vi "Load.vi"(6 "replace if found? (F)":bool, 8 "error in (no error)":errorcluster, 9 "create file if necessary? (T)":bool=TRUE, 10 "configuration file path":path, 11 "DSF Configuration Reference in":T1) -> (0 "error out":errorcluster, 1 "file replaced?":bool, 2 "file created?":bool, 3 "DSF Configuration Reference out":T1)   [LabVIEW 2017, in "Data Sharing Framework Core.lvlib" / "Data Sharing Framework Configuration.lvlib"]
uses:
  Data Sharing Framework Configuration.lvlib
  Controls/Session/DSF Configuration Reference.ctl
  Controls/DSF File Format/Internal.DSF Configuration.ctl
  Public/Controls/DSF Version Info.ctl
  Controls/DSF File Format/Internal.DSF Plugin with ID.ctl
  Controls/DSF File Format/Internal.DSF Plugin Info.ctl
  Public/Controls/DSF Timing Info.ctl
  Controls/DSF File Format/Internal.DSF Group with ID.ctl
  Controls/DSF File Format/Internal.DSF Group Info.ctl
  Controls/DSF File Format/Internal.DSF Transfer with ID.ctl
  Controls/DSF File Format/Internal.DSF Transfer Info.ctl
  Controls/DSF File Format/Internal.DSF Channel with ID.ctl
  Controls/DSF File Format/Internal.DSF Channel Info.ctl
  Controls/DSF File Format/Internal.DSF Settings with ID.ctl
  Controls/DSF File Format/Internal.DSF Settings Info.ctl
  Controls/Session/DSF Config Data.ctl
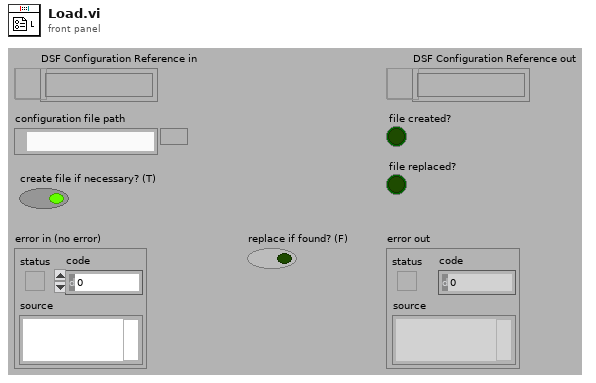
[diagram p1: front panel]
types:
  T1 = typedef "Data Sharing Framework Core.lvlib/Data Sharing Framework Configuration.lvlib/DSF Configuration Reference.ctl" = refnum<data-value>
  T2 = typedef "Data Sharing Framework Core.lvlib/Data Sharing Framework Configuration.lvlib/DSF Config Data.ctl" = cluster{"dsf configuration":T3, "path":path, "dirty":bool}
  T3 = typedef "Data Sharing Framework Core.lvlib/Data Sharing Framework Configuration.lvlib/Internal.DSF Configuration.ctl" = cluster{"dsfversion":T4, "version":T4, "plugins":T5[], "groups":T8[], "transfers":T10[], "channels":T12[], "settings":T14[]}
  T4 = typedef "Data Sharing Framework Core.lvlib/Data Sharing Framework Configuration.lvlib/DSF Version Info.ctl" = cluster{"major":u32, "minor":u32, "fix":u32, "build":string}
  T5 = typedef "Data Sharing Framework Core.lvlib/Data Sharing Framework Configuration.lvlib/Internal.DSF Plugin with ID.ctl" = cluster{"id":string, "values":T6}
  T6 = typedef "Data Sharing Framework Core.lvlib/Data Sharing Framework Configuration.lvlib/Internal.DSF Plugin Info.ctl" = cluster{"type":string, "timing":T7, "group ids":string[], "settings id":string}
  T7 = typedef "Data Sharing Framework Core.lvlib/Data Sharing Framework Configuration.lvlib/DSF Timing Info.ctl" = cluster{"priority":u64, "decimation":u64, "offset":u64}
  T8 = typedef "Data Sharing Framework Core.lvlib/Data Sharing Framework Configuration.lvlib/Internal.DSF Group with ID.ctl" = cluster{"id":string, "values":T9}
  T9 = typedef "Data Sharing Framework Core.lvlib/Data Sharing Framework Configuration.lvlib/Internal.DSF Group Info.ctl" = cluster{"direction":i32, "timing":T7, "transfer ids":string[], "settings id":string}
  T10 = typedef "Data Sharing Framework Core.lvlib/Data Sharing Framework Configuration.lvlib/Internal.DSF Transfer with ID.ctl" = cluster{"id":string, "values":T11}
  T11 = typedef "Data Sharing Framework Core.lvlib/Data Sharing Framework Configuration.lvlib/Internal.DSF Transfer Info.ctl" = cluster{"byte order":i32, "channel ids":string[], "settings id":string}
  T12 = typedef "Data Sharing Framework Core.lvlib/Data Sharing Framework Configuration.lvlib/Internal.DSF Channel with ID.ctl" = cluster{"id":string, "values":T13}
  T13 = typedef "Data Sharing Framework Core.lvlib/Data Sharing Framework Configuration.lvlib/Internal.DSF Channel Info.ctl" = cluster{"count":u64, "buffer offset":u64, "data type":i32, "settings id":string}
  T14 = typedef "Data Sharing Framework Core.lvlib/Data Sharing Framework Configuration.lvlib/Internal.DSF Settings with ID.ctl" = cluster{"id":string, "values":T15}
  T15 = typedef "Data Sharing Framework Core.lvlib/Data Sharing Framework Configuration.lvlib/Internal.DSF Settings Info.ctl" = cluster{"key":string, "value":string}[]
  T16 = enum16{"open", "replace", "create", "open or create", "replace or create", "replace or create with confirmation"}
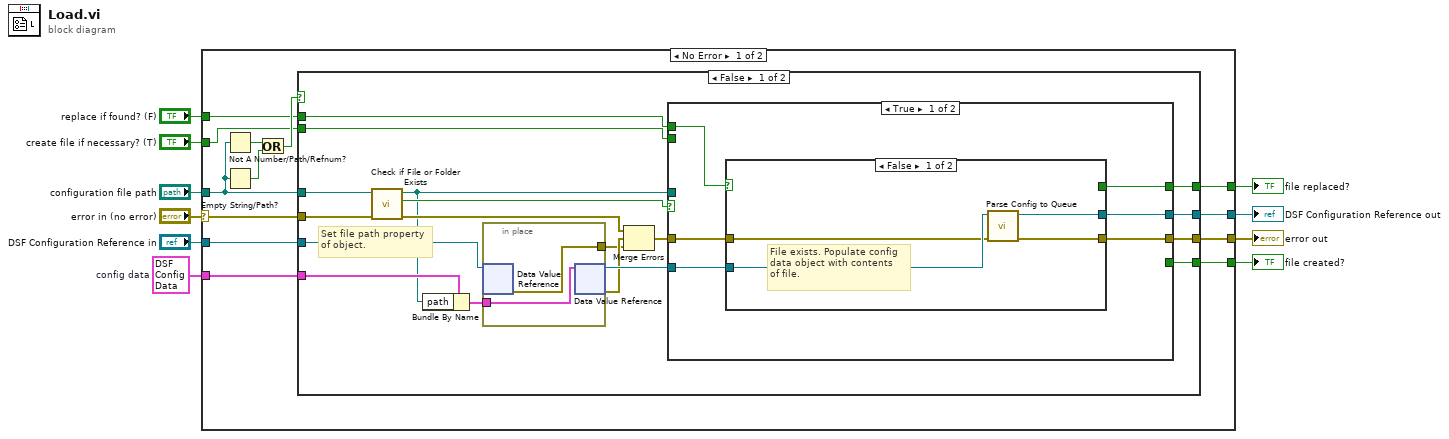
[diagram p0: block diagram]
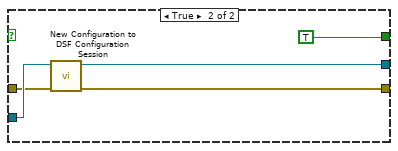
[diagram p2: hidden frame]
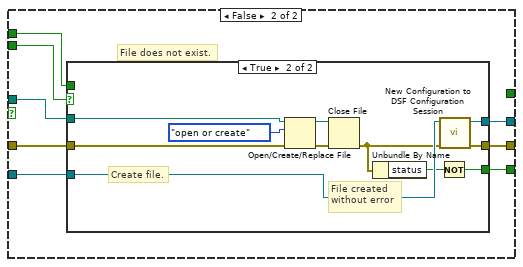
[diagram p3: hidden frame]
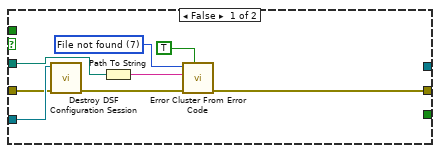
[diagram p4: hidden frame]
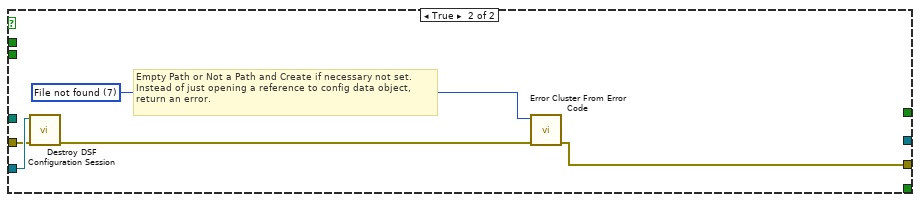
[diagram p5: hidden frame]
diagram:
  w3 = T2 {"dsf configuration"={"dsfversion"={"major"=0, "minor"=0, "fix"=0, "build"=""}, "version"={"major"=0, "minor"=0, "fix"=0, "build"=""}, "plugins"=[], "groups"=[], "transfers"=[], "channels"=[], "settings"=[]}, "path"=path "", "dirty"=FALSE}  # config data
  n1 = case shown="No Error" "error in (no error)" {
    selector: "error in (no error)" -> [w19 w92]
    tunnel: [w16 w92] -> w9
    tunnel: [w17 w91] -> w4
    tunnel: "configuration file path" -> [w18 _]
    tunnel: "create file if necessary? (T)" -> [w20 _]
    tunnel: [w15 _] -> w6
    tunnel: "DSF Configuration Reference in" -> [w14 w91]
    tunnel: w3 -> [w13 _]
    tunnel: "replace if found? (F)" -> [w12 _]
    tunnel: [w11 _] -> w1
    frame No Error {
      n2 = Not A Number/Path/Refnum? ("Not A Number/Path/dsf refnum?")(number/path/refnum=w18) -> (NaN/Path/Refnum?=w22:bool)
      n3 = Empty String/Path?(string/path=w18) -> (empty?=w23:bool)
      n4 = Or(x=w22, y=w23) -> (x .or. y?=w21:bool)
      n5 = case shown="False" w21 {
        tunnel: [w41 w90] -> w16
        tunnel: w18 -> [w36 _]
        tunnel: w20 -> [w40 _]
        tunnel: w19 -> [w34 w87]
        tunnel: [w39 _] -> w17
        tunnel: [w38 _] -> w15
        tunnel: w14 -> [w31 w88]
        tunnel: w13 -> [w35 _]
        tunnel: w12 -> [w25 _]
        tunnel: [w24 _] -> w11
        frame False {
          # "Set file path property\nof object."
          n6 = call <vilib>:"Check if File or Folder Exists.vi"("error in (no error)"=w34, "path"=w36) -> ("error out"=w33:errorcluster, "file or folder exists?"=w37:bool, "dup path"=w32:path)  [unwired: 7 out]
          n7 = Bundle By Name(cluster=w35, "path"=w32) -> (w30:T2)
          n8 = in-place {
            in-place-border: w30 -> [w43]
            in-place-border: [w42] -> w26
            n9 = in-place-dvr #1(w31) -> (w42:errorcluster)  [unwired: 1 out]
            n10 = in-place-dvr #1(w43) -> (w29:T1, w27:errorcluster)
          }
          n11 = Merge Errors(w33, w27, w26) -> (w28:errorcluster)
          n12 = case shown="True" w37 {
            tunnel: [w48 w65] -> w41
            tunnel: w32 -> [_ w66]
            tunnel: w40 -> [_ w64]
            tunnel: w29 -> [w49 w61]
            tunnel: [w47 w62] -> w39
            tunnel: [_ w63] -> w38
            tunnel: w28 -> [w46 w60]
            tunnel: w25 -> [w45 w59]
            tunnel: [w44 _] -> w24
            frame True {
              n13 = case shown="False" w45 {
                tunnel: w49 -> [w53 w56]
                tunnel: [w52 w57] -> w48
                tunnel: [w51 w58] -> w47
                tunnel: w46 -> [w50 w55]
                tunnel: [_ TRUE] -> w44
                frame False {
                  # "File exists. Populate config\ndata object with contents\nof file."
                  n14 = call "Parse Config to Queue.vi"("error in"=w50, "DSF Configuration Session in"=w53) -> ("error out"=w52:errorcluster, "DSF Configuration Session out"=w51:T1)  [unwired: 8 out]
                }
                frame True {
                  n15 = call "New Configuration to DSF Configuration Session.vi"("error in"=w55, "DSF Configuration Session in"=w56) -> ("error out"=w57:errorcluster, "DSF Configuration Session out"=w58:T1)  [unwired: 8 out]
                }
              }
            }
            frame False {
              # "File does not exist."
              n16 = case shown="True" w64 {
                tunnel: w66 -> [w68 w85]
                tunnel: [w73 w79] -> w65
                tunnel: [_ w76] -> w63
                tunnel: [_ w80] -> w62
                tunnel: w61 -> [w72 w81]
                tunnel: w60 -> [w71 w82]
                tunnel: w59 -> [_ _]
                frame False {
                  w74 = u16 7 items=["No error", "Argument error", "Memory is full", "Out of zone", "End of file", "File already open", "Generic file I/O error", "File not found", "File permission error", "Disk is full", "Duplicate path", "Too many files open", "System feature not enabled", "Resource file not found", "Cannot add resource", "Resource not found", "Image not found", "Image memory error", "Pen does not exist", "Config type invalid", "Config token not found", "Config parse error", "Config memory error", "Bad external code format", "Bad external code offset", "External code not present", "Null window", "Destroy window error", "Null menu", "Print aborted", "Bad print record", "Print driver error", "Windows error during printing", "Memory error during printing", "Print dialog error", "Generic print error", "Invalid device refnum", "Device not found", "Device parameter error", "Device unit error", "Cannot open device", "Device call aborted", "Generic error", "Cancelled by user", "Object ID too low", "Object ID too high", "Object not in heap", "Unknown heap", "Unknown object (invalid DefProc)", "Unknown object (DefProc not in table)", "Message out of range", "Invalid (null) method", "Unknown message", "Manager call not supported", "Bad address", "Network operation in progress", "Network operation timed out", "Connection is busy", "Network attribute not supported", "Network error", "Address in use", "System out of memory", "Connection aborted", "Connection refused", "Not connected", "Already connected", "Connection closed", "Initialization error (interapplication manager)", "Bad occurrence", "Wait on unbound occurrence handler", "Occurrence queue overflow", "Datalog type conflict", "Unused", "Unrecognized type (interapplication manager)", "Memory corrupt", "Failed to make temporary DLL", "Old CIN version", "Drag socket not found", "Failed to load drop-object", "Failed to register OLE object", "Failed to release OLE object", "Format specifier type mismatch", "Unknown format specifier", "Too few format specifiers", "Too many format specifiers", "Scan failed", "Newer CIN version", "OLE Convert", "Runtime menu error", "Password tampered", "Unknown error code"]
                  n17 = call "Destroy DSF Configuration Session.vi"("error in (no error)"=w71, "DSF Configuration Session in"=w72) -> ("error out"=w70:errorcluster)  [unwired: 9 in]
                  n18 = Path To String(path=w68) -> (string=w67:string)
                  n19 = call <vilib>:"Error Cluster From Error Code.vi"("show call chain? (False)"=TRUE, "error in (no error)"=w70, "error message (\"\")"=w67, "error code (0)"=w74) -> ("error out"=w73:errorcluster)  [unwired: 5 out]
                }
                frame True {
                  # "File created\nwithout error"
                  # "Create file."
                  n20 = Open/Create/Replace File(file path (use dialog)=w85, error in=w82, operation (0:open)=T16."open or create") -> (refnum out=w83:refnum<file>, error out=w84:errorcluster)  [unwired: 4 out]
                  n21 = Close File(refnum=w83, error in=w84) -> (error out=w77:errorcluster)  [unwired: 1 out]
                  n22 = Unbundle By Name(w77) -> ("status"=w78:bool)
                  n23 = Not(x=w78) -> (.not. x?=w76:bool)
                  n24 = call "New Configuration to DSF Configuration Session.vi"("error in"=w77, "DSF Configuration Session in"=w81) -> ("error out"=w79:errorcluster, "DSF Configuration Session out"=w80:T1)  [unwired: 8 out]
                }
              }
            }
          }
        }
        frame True {
          w89 = u16 7 items=["No error", "Argument error", "Memory is full", "Out of zone", "End of file", "File already open", "Generic file I/O error", "File not found", "File permission error", "Disk is full", "Duplicate path", "Too many files open", "System feature not enabled", "Resource file not found", "Cannot add resource", "Resource not found", "Image not found", "Image memory error", "Pen does not exist", "Config type invalid", "Config token not found", "Config parse error", "Config memory error", "Bad external code format", "Bad external code offset", "External code not present", "Null window", "Destroy window error", "Null menu", "Print aborted", "Bad print record", "Print driver error", "Windows error during printing", "Memory error during printing", "Print dialog error", "Generic print error", "Invalid device refnum", "Device not found", "Device parameter error", "Device unit error", "Cannot open device", "Device call aborted", "Generic error", "Cancelled by user", "Object ID too low", "Object ID too high", "Object not in heap", "Unknown heap", "Unknown object (invalid DefProc)", "Unknown object (DefProc not in table)", "Message out of range", "Invalid (null) method", "Unknown message", "Manager call not supported", "Bad address", "Network operation in progress", "Network operation timed out", "Connection is busy", "Network attribute not supported", "Network error", "Address in use", "System out of memory", "Connection aborted", "Connection refused", "Not connected", "Already connected", "Connection closed", "Initialization error (interapplication manager)", "Bad occurrence", "Wait on unbound occurrence handler", "Occurrence queue overflow", "Datalog type conflict", "Unused", "Unrecognized type (interapplication manager)", "Memory corrupt", "Failed to make temporary DLL", "Old CIN version", "Drag socket not found", "Failed to load drop-object", "Failed to register OLE object", "Failed to release OLE object", "Format specifier type mismatch", "Unknown format specifier", "Too few format specifiers", "Too many format specifiers", "Scan failed", "Newer CIN version", "OLE Convert", "Runtime menu error", "Password tampered", "Unknown error code"]
          # "Empty Path or Not a Path and Create if necessary not set.\nInstead of just opening a reference to config data object,\nreturn an error."
          n25 = call "Destroy DSF Configuration Session.vi"("error in (no error)"=w87, "DSF Configuration Session in"=w88) -> ("error out"=w86:errorcluster)  [unwired: 9 in]
          n26 = call <vilib>:"Error Cluster From Error Code.vi"("error in (no error)"=w86, "error code (0)"=w89) -> ("error out"=w90:errorcluster)  [unwired: 1 in, 6 out]
        }
      }
    }
    frame Error {
    }
  }
  "error out" <- w9
  "file created?" <- w6
  "DSF Configuration Reference out" <- w4
  "file replaced?" <- w1
